vi "Meta Program.vi"() -> ()   [LabVIEW 2018]
panel:
  in  "CB type":u16(ring)=2 items=["1 bpc"=1, "2 bpc"=2, "3 bpc"=3, "4 bpc"=4, "5 bpc"=5]
  in  "Final BL Start":dbl=1.0
  in  "Initial BL Start":dbl=5.0
  in  "BL Start Step":dbl=0.2
  in  "Final SL Start":dbl=1.0
  in  "Initial SL Start":dbl
  in  "SL Start Step":dbl=0.2
  in  "Final WL Step":dbl=0.1
  in  "Initial WL Step":dbl=0.1
  in  "WL Step Step":dbl=0.01
  in  "Final BL Step":dbl=0.42
  in  "Initial BL Step":dbl=5.0
  in  "BL Step Step":dbl=0.08
  in  "Final SL Step":dbl=0.42
  in  "Initial SL Step":dbl=0.02
  in  "SL Step Step":dbl=0.08
  in  "Write Algorithm":u16(ring)=3 items=["Ping-Pong", "ISPP", "FPPV", "SDR"]
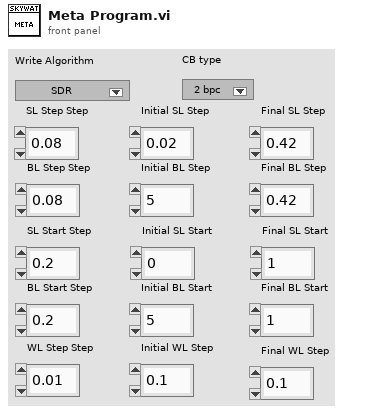
[diagram p1: front panel]
types:
  T1 = enum32{"FORM", "SET", "RESET", "READ", "Sweep", "Target", "CB (W)", "CB (R)", "Cycle"}
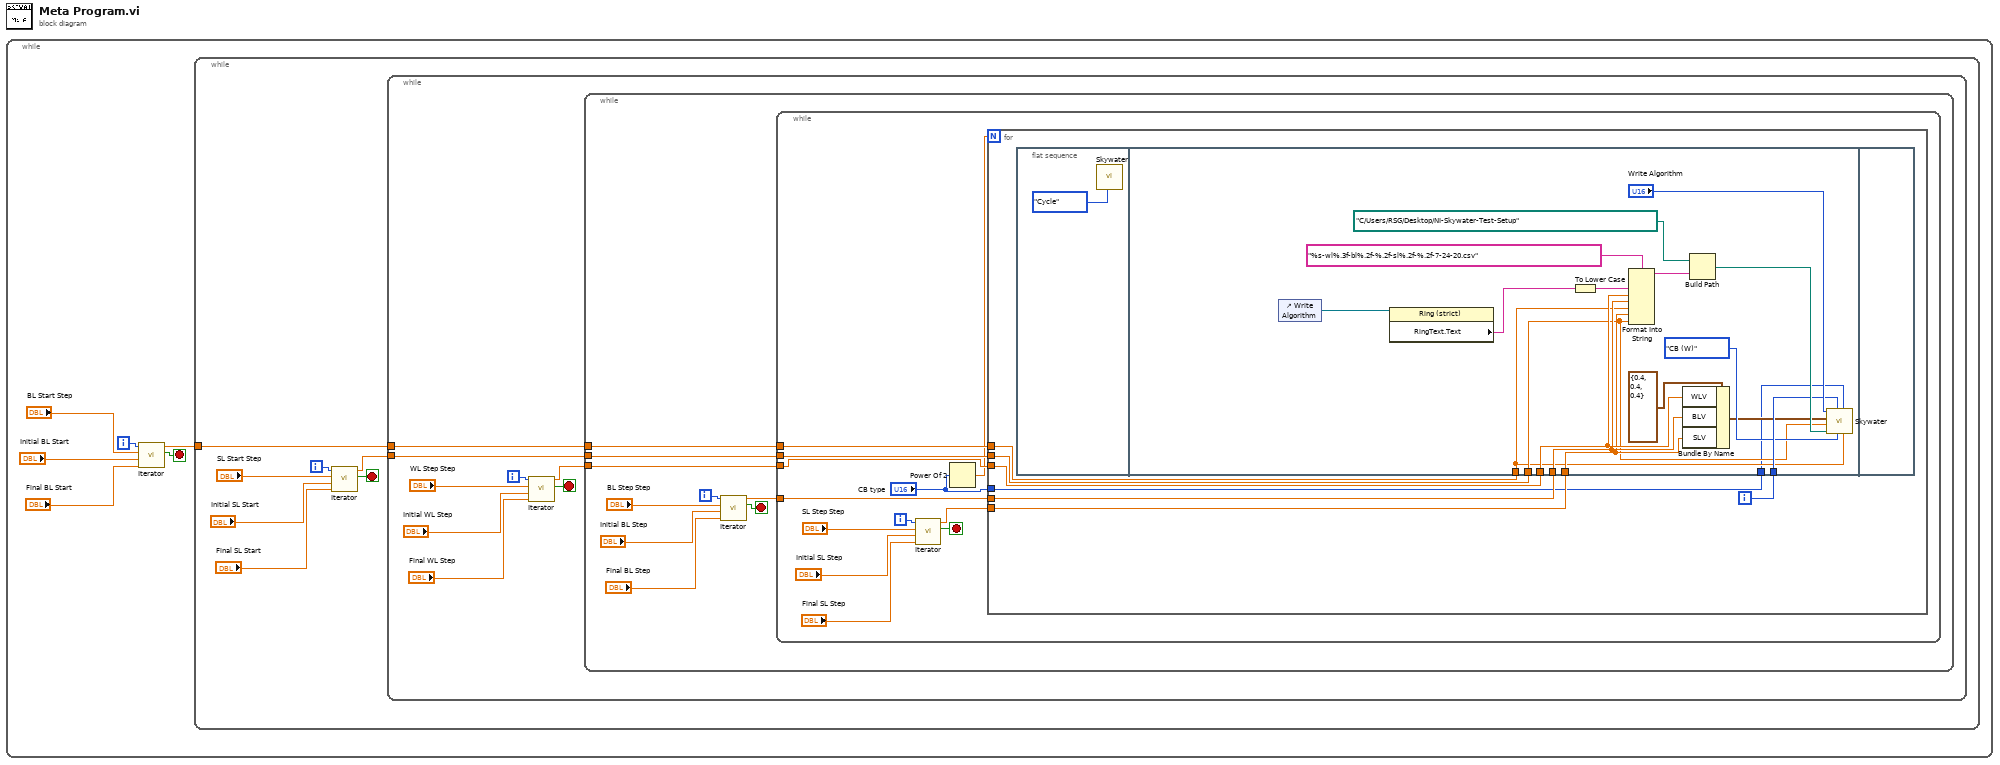
[diagram p0: block diagram]
diagram:
  n1 = while {
    i -> [w5]
    stop <- w2 stop-if-true
    n2 = call "Iterator.vi"("Final Value"="Final BL Start", "Initial Value"="Initial BL Start", "Step"="BL Start Step", "i"=w5) -> ("End Loop"=w2:bool, "Current Value"=w1:dbl)  [unwired: 6 in]
    n3 = while {
      tunnel: w1 -> [w7]
      i -> [w10]
      stop <- w9 stop-if-true
      n4 = call "Iterator.vi"("Final Value"="Final SL Start", "Initial Value"="Initial SL Start", "Step"="SL Start Step", "i"=w10) -> ("End Loop"=w9:bool, "Current Value"=w8:dbl)  [unwired: 6 in]
      n5 = while {
        tunnel: w8 -> [w15]
        tunnel: w7 -> [w14]
        i -> [w18]
        stop <- w17 stop-if-true
        n6 = call "Iterator.vi"("Final Value"="Final WL Step", "Initial Value"="Initial WL Step", "Step"="WL Step Step", "i"=w18) -> ("End Loop"=w17:bool, "Current Value"=w16:dbl)  [unwired: 6 in]
        n7 = while {
          tunnel: w16 -> [w24]
          tunnel: w15 -> [w23]
          tunnel: w14 -> [w22]
          i -> [w27]
          stop <- w26 stop-if-true
          n8 = call "Iterator.vi"("Final Value"="Final BL Step", "Initial Value"="Initial BL Step", "Step"="BL Step Step", "i"=w27) -> ("End Loop"=w26:bool, "Current Value"=w25:dbl)  [unwired: 6 in]
          n9 = while {
            tunnel: w25 -> [w36]
            tunnel: w24 -> [w35]
            tunnel: w23 -> [w34]
            tunnel: w22 -> [w33]
            i -> [w39]
            stop <- w37 stop-if-true
            n10 = call "Iterator.vi"("Final Value"="Final SL Step", "Initial Value"="Initial SL Step", "Step"="SL Step Step", "i"=w39) -> ("End Loop"=w37:bool, "Current Value"=w38:dbl)  [unwired: 6 in]
            n11 = Power Of 2(x="CB type") -> (2^x=w32:dbl)
            n12 = for {
              N: w32 -> [_]
              tunnel: w38 -> [w48]
              tunnel: w36 -> [w47]
              tunnel: w35 -> [w46]
              tunnel: w34 -> [w45]
              tunnel: w33 -> [w44]
              tunnel: "CB type" -> [w43]
              i -> [w49]
              n13 = flat-sequence {
                tunnel: w49 -> [w60]
                tunnel: w48 -> [w54]
                tunnel: w47 -> [w55]
                tunnel: w46 -> [w56]
                tunnel: w45 -> [w53]
                tunnel: w44 -> [w52]
                tunnel: w43 -> [w51]
                frame #0 {
                  n14 = call "Skywater.vi"("Mode"=T1."Cycle") -> ()  [unwired: 11 in]
                }
                frame #1 {
                  n15 = control-ref of="Write Algorithm"() -> (w67:refnum<vi>)
                  n16 = property class="Ring (strict)"(reference=w67) -> ("RingText.Text"=w66:string)  [unwired: 1 in, 2 out]
                  n17 = To Lower Case(string=w66) -> (all lower case string=w61:string)
                  n18 = Format Into String(format string="%s-wl%.3f-bl%.2f-%.2f-sl%.2f-%.2f-7-24-20.csv", w61, w56, w55, w52, w54, w53) -> (resulting string=w63:string)  [unwired: 2 in, 1 out]
                  n19 = Bundle By Name(cluster=cluster{"WLV":dbl, "BLV":dbl, "SLV":dbl} {"WLV"=0.4, "BLV"=0.4, "SLV"=0.4} ("Step Size"), "WLV"=w56, "BLV"=w55, "SLV"=w54) -> (w57:cluster{"WLV":dbl, "BLV":dbl, "SLV":dbl})
                  n20 = Build Path(base path=path "C:/Users/RSG/Desktop/NI-Skywater-Test-Setup", name or relative path=w63) -> (appended path=w64:path)
                  n21 = call "Skywater.vi"("BLV Start"=w52, "CB type"=w51, "Mode"=T1."CB (W)", "CB offset"=w60, "CB write outfile"=w64, "SLV Start"=w53, "Step Size"=w57, "Write Algorithm"="Write Algorithm") -> ()  [unwired: 4 in]
                }
                frame #2 {
                }
              }
            }
          }
        }
      }
    }
  }
